vi "Origin_Export_7_24a_JW.vi"(7 "Analysis Array":string[][](array[string]), 8 "error in (no error)":errorcluster, 9 "Parameter Worksheet Name":string, 10 "Parameter Folder Script":string, 11 "Origin.IOApplication":refnum<k7>) -> (0 "error out":errorcluster, 2 "Origin.Worksheet":refnum<k7>, 3 "reference out":refnum<k7>)   [LabVIEW 2011]
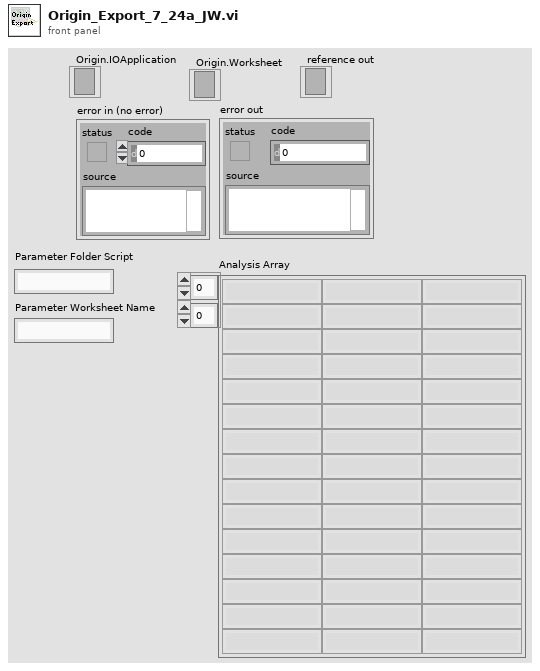
[diagram p1: front panel]
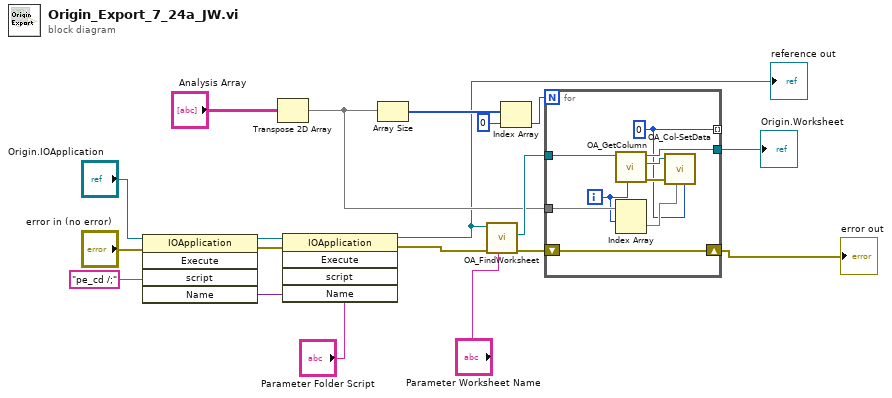
[diagram p0: block diagram]
diagram:
  n1 = invoke class="IOApplication" method="Execute"(reference="Origin.IOApplication", error in="error in (no error)", "script"="pe_cd /;") -> (reference out=w18:refnum<k7>, error out=w17:errorcluster, "Name"=w16:variant)  [unwired: 2 in, 2 out]
  n2 = Transpose 2D Array(2D array="Analysis Array") -> (transposed array=w7:string[][])
  n3 = invoke class="IOApplication" method="Execute"(reference=w18, error in=w17, "script"="Parameter Folder Script", "Name"=w16) -> (reference out=w3:refnum<k7>, error out=w2:errorcluster)  [unwired: 1 in, 3 out]
  "reference out" <- w3
  n4 = Array Size(array=w7) -> (size(s)=w13:i32[])
  n5 = call <userlib>:"OA_FindWorksheet.vi"("Name"="Parameter Worksheet Name", "error in (no error)"=w2, "Origin.IOApplication"=w3) -> ("error out"=w14:errorcluster, "Origin.Worksheet"=w15:refnum<k7>)  [unwired: 6 in, 1 out]
  n6 = Index Array(array=w13, index=0) -> (element=w12:i32)
  n7 = for {
    N: w12 -> [_]
    tunnel: w15 -> [w28]
    tunnel: w7 -> [w27]
    tunnel: [w26] -> w8
    shift-right: [w22] -> w1
    shift-left: w14 -> [w22]
    tunnel: [w20] -> _ mode=indexing
    i -> [w21]
    w20 = 0
    n8 = call <userlib>:"OA_GetColumn.vi"("Column Name/Index"=w21, "Origin.Worksheet"=w28) -> ("error out"=w24:errorcluster, "Origin.Column"=w25:refnum<k7>, "Origin.Worksheet"=w26:refnum<k7>)  [unwired: 7 in]
    n9 = Index Array(array=w27, index (row)=w21) -> (element=w23:string[])  [unwired: 1 in]
    n10 = call <userlib>:"OA_Col-SetData.vi"("Origin.Column"=w25, "error in (no error)"=w24, "data"=w23, "nOffset"=w20) -> ()  [unwired: 3 in, 3 out]
  }
  "Origin.Worksheet" <- w8
  "error out" <- w1
